vi "确定波特率.vi"(1 "GPRS参数":i32 format="%x") -> (0 "波特率":i32)   [LabVIEW 2015]
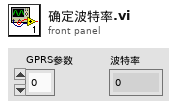
[diagram p1: front panel]
types:
  T1 = typedef "GPRS波特率参数.ctl" = i32[]
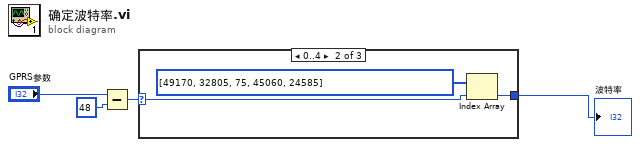
[diagram p0: block diagram]
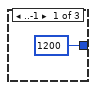
[diagram p2: hidden frame]
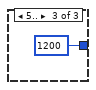
[diagram p3: hidden frame]
diagram:
  n1 = Subtract(x="GPRS参数", y=u16 48) -> (x-y=w2:i32)
  n2 = case shown="0..4" w2 {
    selector: w2 -> [_ w7 _]
    tunnel: [1200 w6 1200] -> w1
    frame ..-1 {
    }
    frame 0..4 {
      n3 = Index Array(array=T1 [49170, 32805, 75, 45060, 24585], index=w7) -> (element=w6:i32)
    }
    frame 5.. {
    }
  }
  "波特率" <- w1
